vi "Matrix_plot.vi"() -> ()   [LabVIEW 2018]
panel:
  out "x = y?":bool
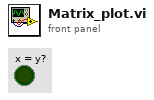
[diagram p1: front panel]
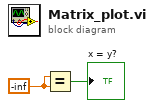
[diagram p0: block diagram]
diagram:
  w2 = -inf
  n1 = Equal?(x=w2, y=w2) -> (x = y?=→"x = y?":bool)
